vi "Read Frame Data.vi"(8 "error in (no error)":errorcluster, 11 "BML Pattern Creater in":refnum<class "BML Pattern Creater.lvclass">) -> (0 "error out":errorcluster, 2 "Frame Data":T1={"Pattern_Name"="", "Data"=[], "Start_Addr"=0, "ChipID"=1, "num of wait ms"=0, "Opcode"=[], "BML OM"=enum."Normal", "BurstLength"=enum."0", "FSN"=0, "R/W?"=enum."Read"} {"Start_Addr" format="%x"; "Data" format="%x"}, 3 "BML Pattern Creater out":refnum<class "BML Pattern Creater.lvclass">)   [LabVIEW 2018, in "BML Pattern Creater.lvlib" / "BML Pattern Creater.lvclass"]
uses:
  BML Pattern Creater.lvclass
  Ctls/FRM Data - BML.ctl
  Ctls/OM - BML.ctl
  Ctls/Burst Length.ctl
  Ctls/RW Options.ctl
  BML Pattern Creater.lvclass/BML Pattern Creater.ctl
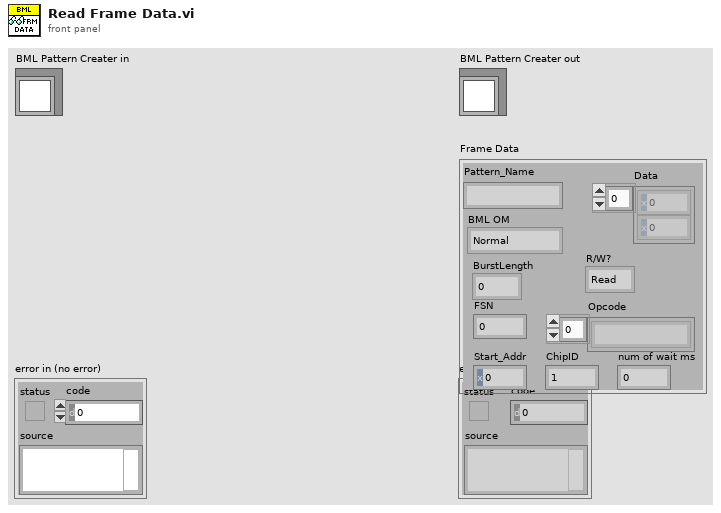
[diagram p1: front panel]
types:
  T1 = typedef "FRM Data - BML.ctl" = cluster{"Pattern_Name":string, "Data":u8[], "Start_Addr":u16, "ChipID":u8, "num of wait ms":i8, "Opcode":string[], "BML OM":T2, "BurstLength":T3, "FSN":u8, "R/W?":T4}
  T2 = typedef "OM - BML.ctl" = enum16{"Normal", "ImmeEffect", "InitSlaveID", "LoadData"}
  T3 = typedef "Burst Length.ctl" = enum8{"0", "2", "3", "4", "5", "8", "16", "32"}
  T4 = typedef "RW Options.ctl" = enum16{"Read", "Write", "R/W"}
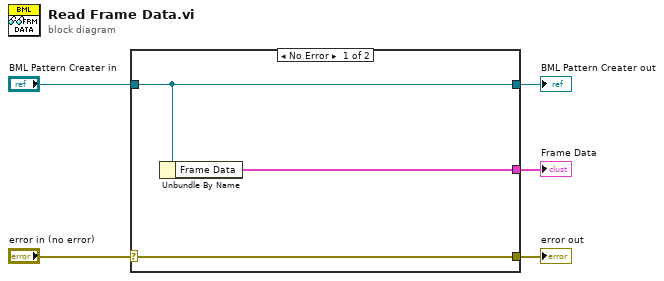
[diagram p0: block diagram]
diagram:
  n1 = case shown="No Error" "error in (no error)" {
    selector: "error in (no error)" -> [w8 w9]
    tunnel: [w8 w9] -> w4
    tunnel: [w7 w10] -> w2
    tunnel: "BML Pattern Creater in" -> [w7 w10]
    tunnel: [w6 _] -> w1
    frame No Error {
      n2 = Unbundle By Name(w7) -> ("Frame Data"=w6:T1)
    }
    frame Error {
    }
  }
  "error out" <- w4
  "BML Pattern Creater out" <- w2
  "Frame Data" <- w1
